vi "GenerateBurst.vi"(8 "error in (no error)":errorcluster, 9 "Burst mode":T1, 11 "reference in":refnum<class "sim_MmW.lvclass">) -> (0 "error out":errorcluster, 3 "reference out":refnum<class "sim_MmW.lvclass">)   [LabVIEW 2019, in "sim_MmW.lvclass"]
doc: "Generates single burst"
uses:
  sim_MmW.lvclass
  C:/Barkhausen mmWave radar/Development/LV/Barkhausen mmWave hardware control/Host/SubVIs/mmWave instrument_class/mmWave instrument.lvclass
  mmWave instrument_class/BurstMode.ctl
  mmWave HW Control/HW custom error.ctl
  mmWave instrument_class/Instrument state.ctl
  mmWave HW Control/mmWave HW Control.lvlib
  mmWave instrument_class/mmWave instrument.lvclass
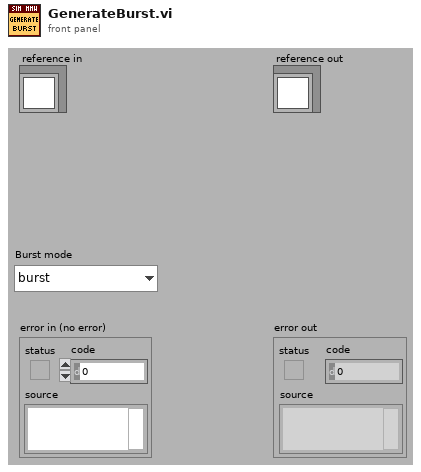
[diagram p1: front panel]
types:
  T1 = typedef "mmWave instrument.lvclass/BurstMode.ctl" = enum16{"burst", "continuous"}
  T2 = typedef "mmWave instrument.lvclass/Instrument state.ctl" = enum16{"Off", "Initialization", "Configuration", "Running", "Calibration"}
  T3 = typedef "mmWave HW Control.lvlib/HW custom error.ctl" = u16
  T4 = typedef "sim_MmW.lvclass/ObjectAttributesRef.ctl" = refnum<data-value>
  T5 = typedef "sim_MmW.lvclass/ObjectAttributes.ctl" = cluster{"RF config":T6, "RX samples":i32, "Downloaded Bursts":map{string, refnum<class "mmWave data.lvclass">}, "TX Fs":dbl, "RX Fs":dbl, "burst sequence":string[], "Burst mode":T1}
  T6 = typedef "mmWave HW Control.lvlib/HW TXRX RF config cluster.ctl" = cluster{"TX.Frequency":dbl, "TX.Gain":dbl, "TX.mmWave adapter":string, "RX.Frequency":dbl, "RX.Gain":dbl, "RX.mmWave adapter":string}
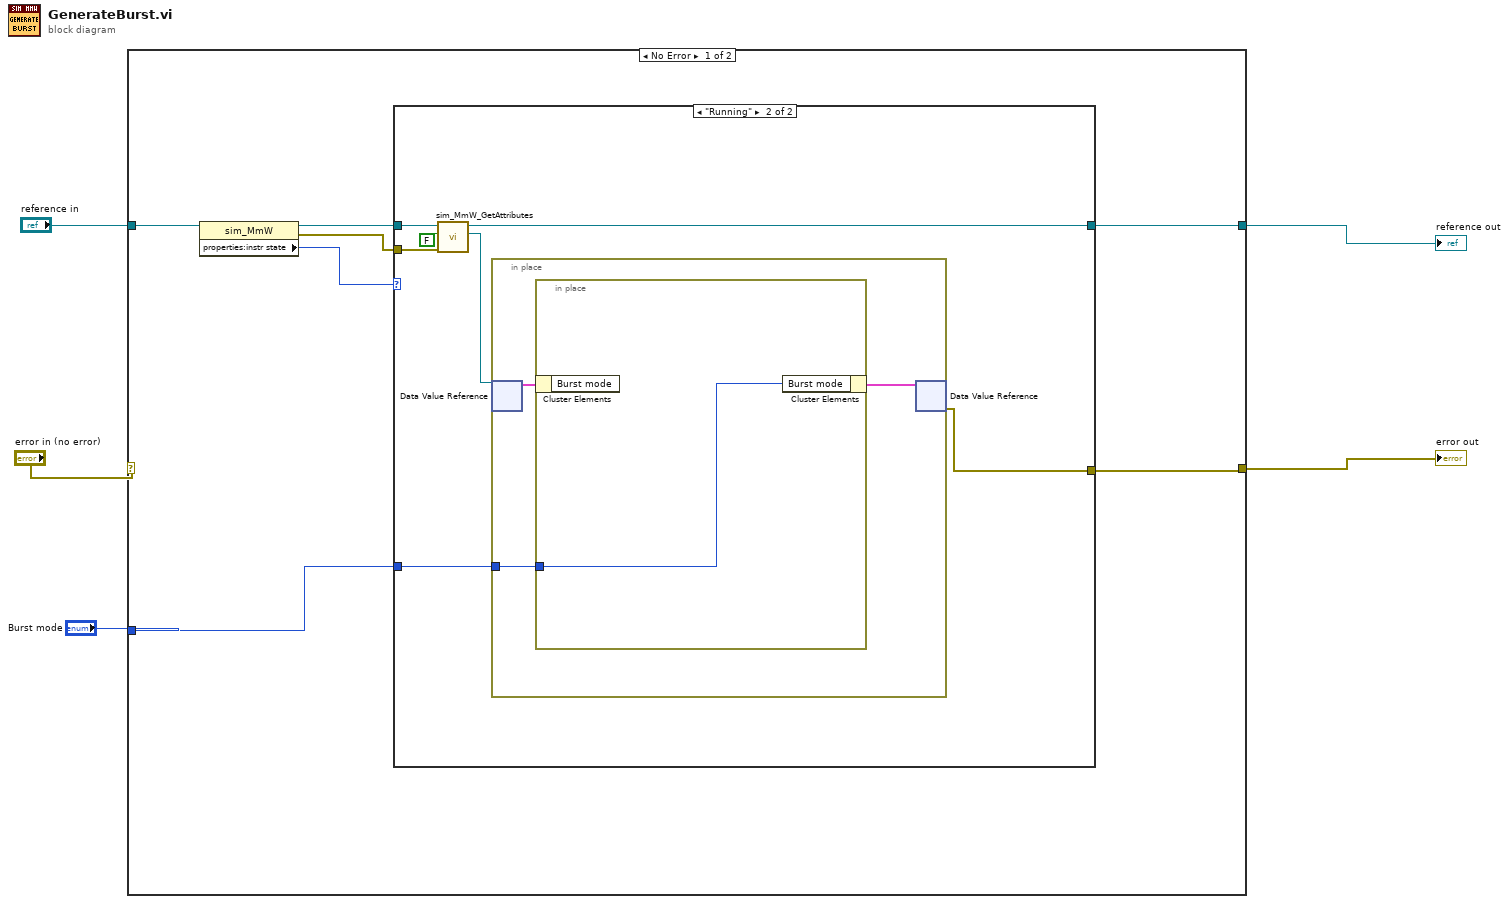
[diagram p0: block diagram]
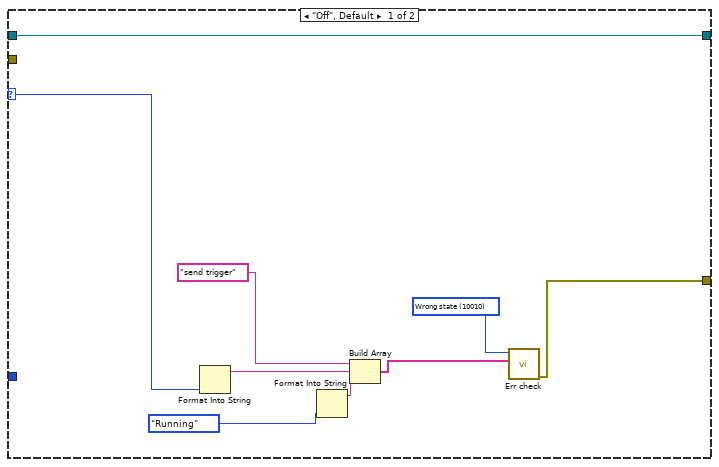
[diagram p2: hidden frame]
diagram:
  n1 = case shown="No Error" "error in (no error)" {
    selector: "error in (no error)" -> [_ w34]
    tunnel: [w7 w34] -> w4
    tunnel: [w11 w33] -> w2
    tunnel: "reference in" -> [w12 w33]
    tunnel: "Burst mode" -> [w6 _]
    frame No Error {
      n2 = property class="sim_MmW"(reference=w12) -> (reference out=w10:refnum<class "sim_MmW.lvclass">, error out=w9:errorcluster, "properties:instr state"=w8:T2)  [unwired: 1 in]
      n3 = case shown="\"Running\"" w8 {
        selector: w8 -> [w14 _]
        tunnel: [w21 w27] -> w11
        tunnel: w10 -> [w21 w25]
        tunnel: w9 -> [_ w24]
        tunnel: [w13 w23] -> w7
        tunnel: w6 -> [_ w22]
        frame "Off", Default {
          w20 = T3 10010 items=["TX list"=10000, "TX length"=10001, "RX length"=10002, "Fs"=10003, "RF Fc"=10004, "Wrong state"=10010] ("HW custom err")
          n4 = Format Into String(w14) -> (resulting string=w18:string)  [unwired: 3 in, 1 out]
          n5 = Format Into String(Instrument_state."Running" ("properties:instr state")) -> (resulting string=w15:string)  [unwired: 3 in, 1 out]
          n6 = Build Array("send trigger", w18, w15) -> (w17:string[])
          n7 = call "Err check.vi"("Variant Control"=w17, "HW custom err"=w20) -> ("error out"=w13:errorcluster)  [unwired: 9 in]
        }
        frame "Running" {
          n8 = call "sim_MmW_GetAttributes.vi"("error in (no error)"=w24, "return data? (T)"=FALSE, "reference in"=w25) -> ("attributes ref"=w26:T4, "reference out"=w27:refnum<class "sim_MmW.lvclass">)  [unwired: 5 in, 2 out]
          n9 = in-place {
            in-place-border: w22 -> [w29]
            n10 = in-place-dvr #1(w26) -> (w30:T5)  [unwired: 1 out]
            n11 = in-place {
              in-place-border: w29 -> [w32]
              n12 = in-place-cluster #2(w30) -> ()  [unwired: 1 out]
              n13 = in-place-cluster #2("Burst mode"=w32) -> (w31:T5)
            }
            n14 = in-place-dvr #1(w31) -> (w23:errorcluster)  [unwired: 1 out]
          }
        }
      }
    }
    frame Error {
    }
  }
  "error out" <- w4
  "reference out" <- w2
